vi "Huber Test Program.vi"() -> ()   [LabVIEW 2018, in "Huber Unistat 410 TCU.lvlib"]
uses:
  Huber Unistat 410 TCU.lvlib
  Huber Unistat 410 Settings.ctl
panel:
  out "Temperature":i32
  in  "Internal?":bool
  out "Running":bool
  out "Connection Error":bool
  in  "stop":bool
  in  "Temp":dbl
  in  "Run":bool
  out "error out":errorcluster
  in  "error in (no error)":errorcluster
  out "Huber Settings":T1
  in  "Huber Settings":T1
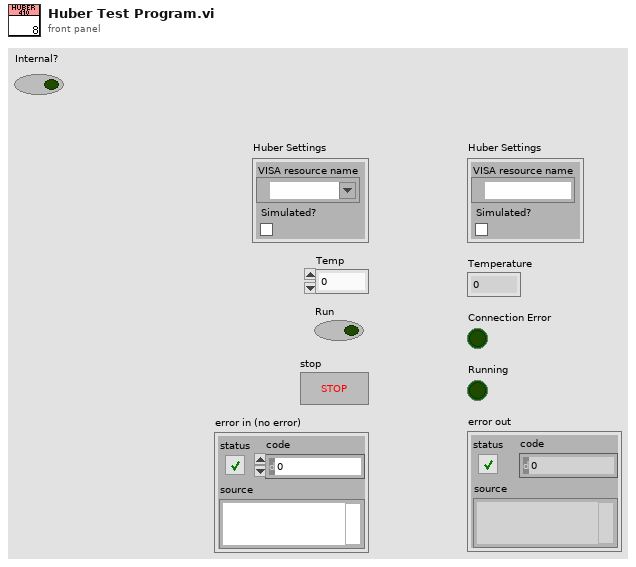
[diagram p1: front panel]
types:
  T1 = typedef "Huber Unistat 410 TCU.lvlib/Huber Unistat 410 Settings.ctl" = cluster{"VISA resource name":refnum<visa-resource-name>, "Simulated?":bool}
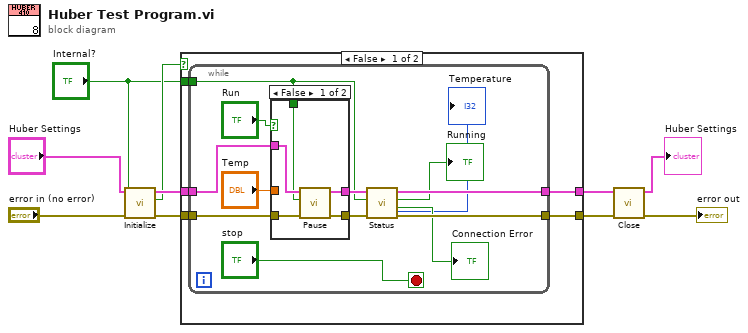
[diagram p0: block diagram]
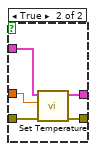
[diagram p2: hidden frame]
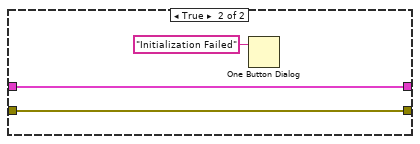
[diagram p3: hidden frame]
diagram:
  n1 = call "Initialize.vi"("error in (no error)"="error in (no error)", "Internal?"="Internal?", "Huber Settings"="Huber Settings") -> ("error out"=w3:errorcluster, "Connection Error"=w2:bool, "Huber Settings"=w4:T1)  [unwired: 6 in]
  n2 = case shown="False" w2 {
    tunnel: [w15 w40] -> w8
    tunnel: [w14 w39] -> w6
    tunnel: w4 -> [w13 w40]
    tunnel: w3 -> [w12 w39]
    tunnel: "Internal?" -> [w11 _]
    frame False {
      n3 = while {
        tunnel: [w28] -> w15
        tunnel: [w27] -> w14
        tunnel: w13 -> [w25]
        tunnel: w12 -> [w24]
        tunnel: w11 -> [w16]
        stop <- "stop" stop-if-true
        n4 = case shown="False" "Run" {
          tunnel: w25 -> [w33 w38]
          tunnel: w24 -> [w32 w37]
          tunnel: [w31 w36] -> w23
          tunnel: [w30 w35] -> w22
          tunnel: "Temp" -> [_ w34]
          tunnel: w16 -> [w29 _]
          frame False {
            n5 = call "Pause.vi"("error in (no error)"=w32, "Internal?"=w29, "Huber Settings"=w33) -> ("error out"=w31:errorcluster, "Huber Settings"=w30:T1)  [unwired: 7 in]
          }
          frame True {
            n6 = call "Set Temperature.vi"("error in (no error)"=w37, "Setpoint"=w34, "Huber Settings"=w38) -> ("error out"=w36:errorcluster, "Huber Settings"=w35:T1)  [unwired: 6 in, 1 out]
          }
        }
        n7 = call "Status.vi"("error in (no error)"=w23, "Internal?"=w16, "Huber Settings"=w22) -> ("error out"=w27:errorcluster, "Connection Error"=→"Connection Error":bool, "Running"=→"Running":bool, "Huber Settings"=w28:T1, "Temperature"=→"Temperature":i32)  [unwired: 4 in]
      }
    }
    frame True {
      n8 = One Button Dialog(message="Initialization Failed") -> ()  [unwired: 1 in, 1 out]
    }
  }
  n9 = call "Close.vi"("error in (no error)"=w6, "Huber Settings"=w8) -> ("error out"=→"error out":errorcluster, "Huber Settings"=→"Huber Settings":T1)  [unwired: 8 in]
